vi "MainNR.vi"(10 "JQMHStartup.lvclass":refnum<class "ModuleStartup.lvclass">, 11 "JQMHCore in":refnum<class "Module.lvclass">) -> ()   [LabVIEW 2024, in "Module.lvclass"]
uses:
  Module.lvclass
  Module.lvclass/Module.ctl
  Startup/ModuleStartup.lvclass
  Startup/Command.ctl
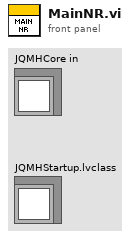
[diagram p1: front panel]
types:
  T1 = typedef "ModuleStartup.lvclass/Command.ctl" = enum16{"Default", "No Override", "Error", "ACK Created", "ACK Mod Reg", "ACK Caller Reg"}
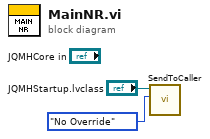
[diagram p0: block diagram]
diagram:
  n1 = call "SendToCaller.vi"("Command"=Command."No Override", "JQMHStartup in"="JQMHStartup.lvclass") -> ()  [unwired: 8 in, 2 out]
